vi "SetVoltageLimit.vi"(2 "error in (no error)":errorcluster, 3 "Voltage":dbl, 4 "Preset":enum16{"0", "1", "2", "3", ""}(ring), 5 "VISA resource name":refnum<visa-resource-name>) -> (0 "error out":errorcluster, 1 "VISA resource name out":refnum<visa-resource-name>)   [LabVIEW 2019, in "9103Series.lvlib"]
uses:
  <instrlib>/9103Series/9103Series.lvlib
panel:
  out "ok?":string
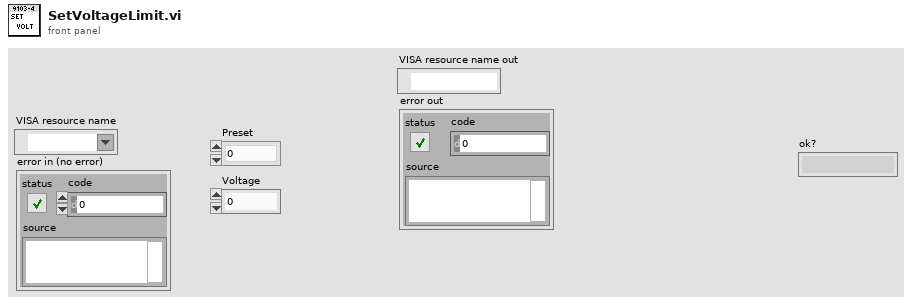
[diagram p1: front panel]
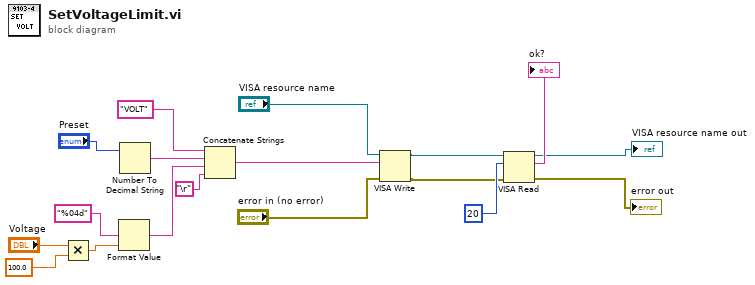
[diagram p0: block diagram]
diagram:
  n1 = Multiply(x="Voltage", y=100.0) -> (x*y=w8:dbl)
  n2 = Format Value(format string="%04d", value (0)=w8) -> (output string=w14:string)  [unwired: 1 in]
  n3 = Number To Decimal String(number="Preset") -> (decimal integer string=w15:string)  [unwired: 1 in]
  n4 = Concatenate Strings("VOLT" ("string"), w15, w14, "\r") -> (w11:string)
  n5 = VISA Write(VISA resource name="VISA resource name", write buffer=w11, error in (no error)="error in (no error)") -> (VISA resource name out=w2:refnum<visa-resource-name>, error out=w1:errorcluster)  [unwired: 1 out]
  n6 = VISA Read(VISA resource name=w2, byte count=u32 20, error in (no error)=w1) -> (VISA resource name out=→"VISA resource name out":refnum<visa-resource-name>, read buffer=→"ok?":string, error out=→"error out":errorcluster)  [unwired: 1 out]
